vi "MU create Calibration.vi"(8 "error in (no error)":errorcluster, 11 "revisionCode":u8) -> (0 "error out":errorcluster, 3 "CalibrationHandle":T1)   [LabVIEW 2017, in "MU_3SL_interface.lvlib"]
doc: "MU_PUBLIC MU_Error MU_setCalibration(MU_Handle handle, const MU_Calibration* calibration);"
uses:
  MU_3SL_interface.lvlib
  handles/CalibrationHandle.ctl
  lib/MU_3SL_interface.dll
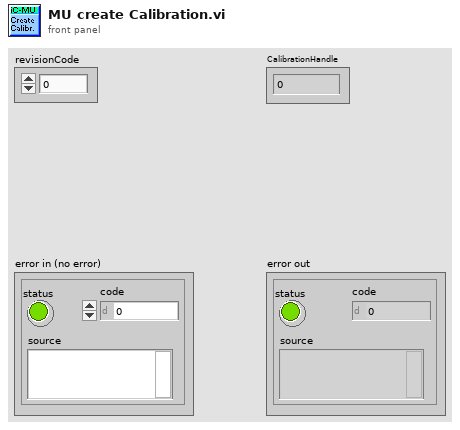
[diagram p1: front panel]
types:
  T1 = typedef "MU_3SL_interface.lvlib/CalibrationHandle.ctl" = u64
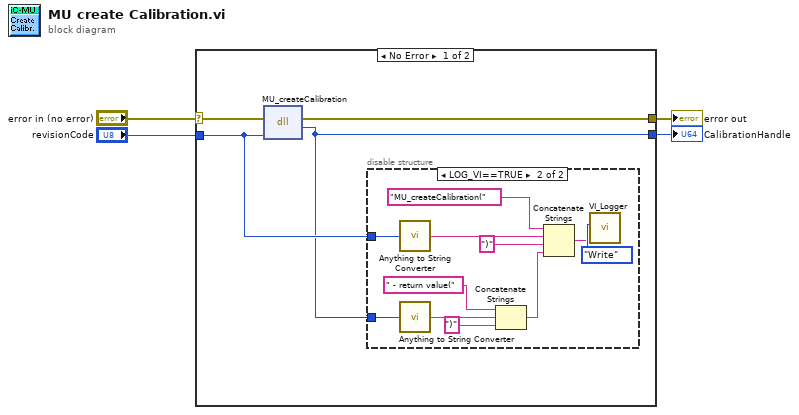
[diagram p0: block diagram]
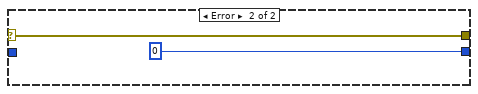
[diagram p3: hidden frame]
diagram:
  n1 = case shown="No Error" "error in (no error)" {
    selector: "error in (no error)" -> [w8 w21]
    tunnel: [w6 u64 0 ("return type")] -> w1
    tunnel: [w5 w21] -> w4
    tunnel: "revisionCode" -> [w7 _]
    frame No Error {
      n2 = dll-call lib="C:/Users/bes/AppData/Roaming/work/mu_9so/icsubmodules/soft_mu_3sl_master/lv_interface/lib/MU_3SL_interface**.*" fn="MU_createCalibration"(error in=w8, "revisionCode"=w7) -> (error out=w5:errorcluster, "return type"=w6:u64)  [unwired: 3 in, 1 out]
      n3 = disable-structure shown="LOG_VI==TRUE" {
        disable-tunnel: w6 -> [_ w15]
        disable-tunnel: w7 -> [_ w10]
        frame condition #0 {
        }
        frame condition #1 (active) {
          n4 = call "Anything to String Converter.vi"("anything"=w10) -> ("String"=w11:string)
          n5 = call "Anything to String Converter.vi"("anything"=w15) -> ("String"=w14:string)
          n6 = Concatenate Strings(" - return value(" ("string"), w14, ")" ("string")) -> (w12:string)
          n7 = Concatenate Strings("MU_createCalibration(" ("Info in"), w11, ")" ("string"), w12) -> (w17:string)
          n8 = call "VI_Logger.vi"("Action (Read)"=enum16{"Write", "Read"}."Write", "Info in"=w17) -> ()  [unwired: 8 in, 2 out]
        }
      }
    }
    frame Error {
    }
  }
  "error out" <- w4
  "CalibrationHandle" <- w1
